vi "Range Minimum Read.vi"(4 "error in (no error)":errorcluster, 6 "Container State":T3, 7 "Display State In":T1) -> (0 "error out":errorcluster, 2 "Value":sgl, 3 "Display State Out":T1)   [LabVIEW 2020, in "3D Pie.xctl"]
uses:
  <vilib>/Math Plots/3D Math Plots/3D Pie/3D Pie XCtrl/3D Pie.xctl
  <vilib>/_xctls/Container State.ctl
  <vilib>/Math Plots/3D Math Plots/3D Pie/3D Pie XCtrl/State.ctl
  <vilib>/Math Plots/3D Math Plots/3D Pie/3D Pie/3D Pie.lvclass
  e:/builds/penguin/labview/branches/2020/dev/dist/vi.lib/Math Plots/3D Math Plots/3D Plot/3D Plot/3D Plot.lvclass
  <vilib>/Math Plots/3D Math Plots/3D Plot/Action String/3DMathPlot Ctrl Act Queue.ctl
  <vilib>/Math Plots/3D Math Plots/3D Plot/Action String/3DMathPlot Ctrl Act Cluster.ctl
  <vilib>/Math Plots/3D Math Plots/3D Plot/Action String/3DMathPlot State Class.ctl
  <vilib>/Math Plots/3D Math Plots/3D Plot/3D Plot/3D Plot.lvclass
  <vilib>/_xctls/XControlSupport.lvlib
panel:
  # "Replace the Value Indicator below with an Indicator of desired type.\nDo not remove this Indicator or the others from the connector pane. \nDo not change the connector pane pattern.\nThe Value Indicator should always be the second terminal from top on the output side in the connector pane."
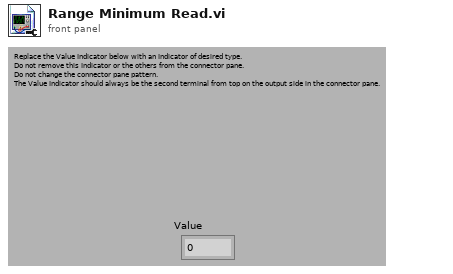
[diagram p1: front panel]
types:
  T1 = typedef "3D Pie.xctl/State.ctl" = cluster{"3D Pie.lvclass":refnum<class "3D Pie.lvclass">, "Control Ref Queue":T2, "Plot Width":u32, "Main Frame Color":u32, "Ramp Palette Color":u32, "Projection Palette Color":u32}
  T2 = typedef "3DMathPlot Ctrl Act Queue.ctl" = refnum<queue>
  T3 = typedef "XControlSupport.lvlib/Container State.ctl" = cluster{"Indicator?":bool, "Run Mode?":bool, " Refnum":refnum<vi>}
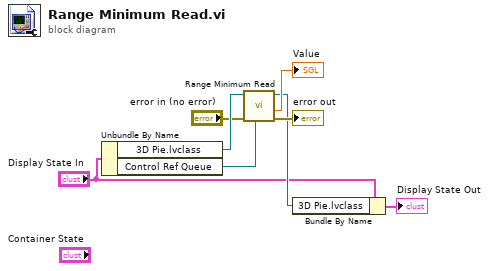
[diagram p0: block diagram]
diagram:
  n1 = Unbundle By Name("Display State In") -> ("3D Pie.lvclass"=w8:refnum<class "3D Pie.lvclass">, "Control Ref Queue"=w1:T2)
  n2 = call <vilib>:"Range Minimum Read.vi"("Control Ref Queue"=w1, "error in (no error)"="error in (no error)", "3D Plot.lvclass in"=w8) -> ("error out"=→"error out":errorcluster, "Range Min"=→"Value":sgl, "3D Plot.lvclass out"=w4:refnum<class "3D Pie.lvclass">)  [unwired: 6 out]
  n3 = Bundle By Name(cluster="Display State In", "3D Pie.lvclass"=w4) -> (→"Display State Out":T1)
